vi "LIA Test CORDIC Host.vi"() -> ()   [LabVIEW 2017]
uses:
  <vilib>/userdefined/Silver/nirio_resource_slv.ctl
  <vilib>/FPGAPlugInAG/PXIe-7976R/niLvFpga_Open_PXIe-7976R.vi
  <vilib>/rvi/interface/common/dynamic/niFpgaDynamicAddResources.vi
  <vilib>/Utility/error.llb/Error Cluster From Error Code.vi
  <vilib>/rvi/errors/niLvFpgaAdjustHostInterfaceError.vi
  <vilib>/rvi/interface/common/niFpgaWaitOnOcc.vi
  <instrlib>/_niInstr/Streaming/v1/Host/Public/Start Finite Stream.vi
  <instrlib>/_niInstr/Streaming/v1/Host/Public/Wait for Stream.vi
  <vilib>/measure/maspectr.llb/FFT Power Spectrum and PSD for 1 Chan (CDB).vi
  <vilib>/FPGAPlugInAG/Dynamic/niLvFpga_Close_Dynamic.vi
  <vilib>/rvi/interface/nirviOpenFPGA/nirviOpenFPGA.xnode
  FPGA Bitfiles/LIA Test Frequency Shift.lvbitx
  <vilib>/rvi/interface/nirviReadWriteControl/nirviReadWriteControl.xnode
  <vilib>/rvi/interface/nirviMethod/nirviMethod.xnode
  <vilib>/rvi/interface/nirviCloseFPGA/nirviCloseFPGA.xnode
  <vilib>/rvi/errors/niLvFpgaMergeErrorWithErrorCode.vi
  <instrlib>/_niInstr/Streaming/v1/Host/niInstr Streaming v1 Host.lvlib
  <vilib>/rvi/interface/Simulation/niFpgaSimulationCallBeginRW.vi
  NiFpgaLv.dll
  <vilib>/measure/NI_MAPro.lvlib
  <vilib>/Analysis/NI_AALBase.lvlib
  <vilib>/FPGAPlugInAG/Dynamic/niLvFpga_StopFifo_Dynamic.vi
  <vilib>/FPGAPlugInAG/Dynamic/niLvFpga_ConfigureFifo_Dynamic.vi
  <vilib>/FPGAPlugInAG/Dynamic/niLvFpga_StartFifo_Dynamic.vi
  Program Files (x86)/National Instruments/LabVIEW 2017/examples/Lock-In Amplifier/lib/host/Lock-In Amplifier Example Host.lvlib
  <vilib>/FPGAPlugInAG/Dynamic/niLvFpga_ReadFifo_Dynamic.vi
panel:
  in  "Stop Button":bool
  in  "Output Frequency":dbl format="%#_p"
  out "standard deviation":dbl format="%0.2p"
  out "mean":dbl format="%.5p"
  out "output sample rate 0":fxp<+,48,1> format="%.48g"
  in  "Decimation":u32
  out "frequency shift rdi count":u64
  out "FIFO rdi count":u64
  in  "Frequency Shift(Hz)":dbl format="%#_p"
  out "Actual Depth":u32 format="%.0p"
  out "Power Specturm Graph":cluster{"f0":dbl, "df":dbl, "magnitude":dbl[]}[](graph)
  out "frequency shift":fxp<+/-,48,0> format="%.48g"
  out "nco frequency 0":fxp<+/-,48,0> format="%.48g"
  in  "NCO Frequency (Hz)":dbl=1000000.0 format="%#_p"
  out "Waveform Graph IQ":dbl[][](graph)
  in  "Number of Elements":u32=10000
  out "error out":errorcluster
  in  "error in":errorcluster
  in  "Resource Name":T1="PXI2Slot2"
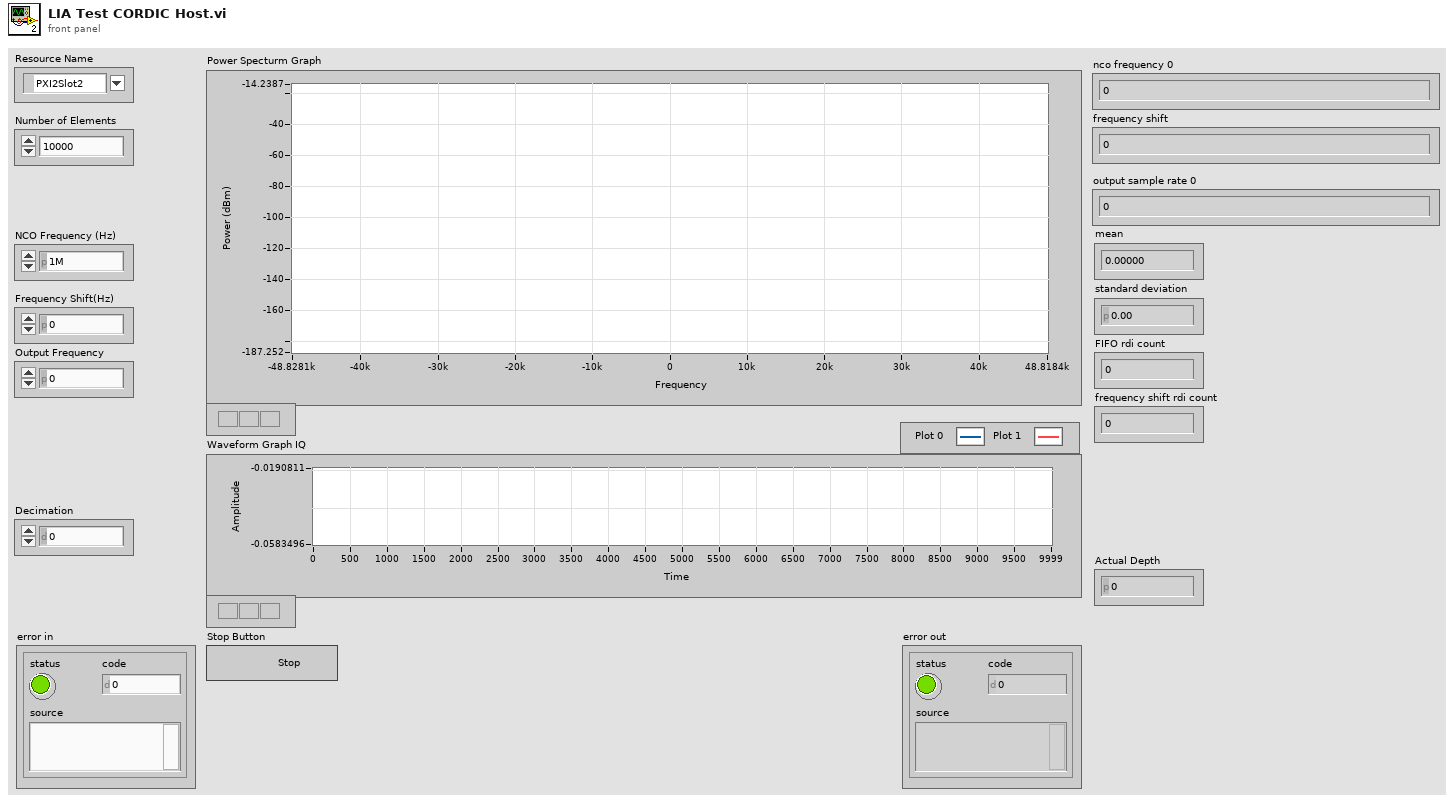
[diagram p1: front panel]
types:
  T1 = typedef "nirio_resource_slv.ctl" = tag
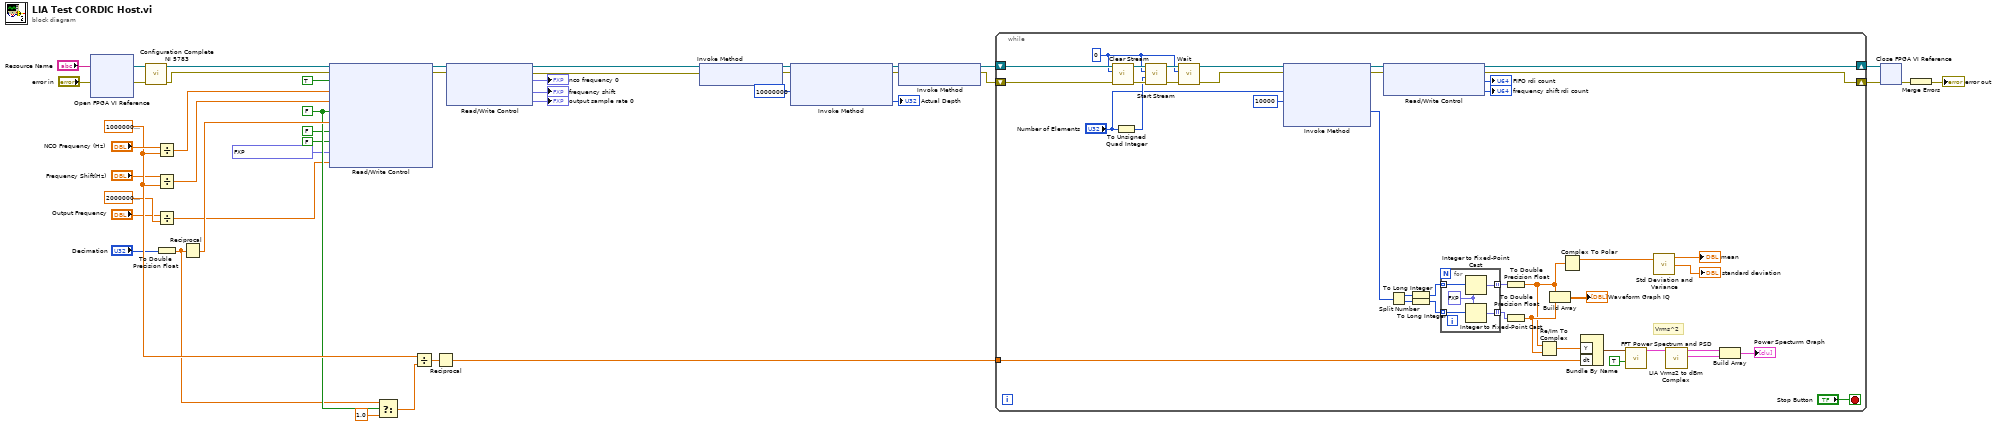
[diagram p0: block diagram]
diagram:
  w27 = 100000000.0 ("Sampling Rate (Hz)")
  w21 = FALSE ("fractional decimator 0 (F)")
  n1 = xnode "Open FPGA VI Reference"("error in"="error in", "resource name"="Resource Name") -> ("FPGA VI Reference Out"=w8:refnum<k20>, "error out"=w7:errorcluster)
  n2 = call "Configuration Complete NI 5783.vi"("error in"=w7, "fpga session in"=w8) -> ("error out"=w6:errorcluster, "fpga session out"=w5:refnum<k20>)  [unwired: 7 in, 1 out]
  n3 = Divide(x="NCO Frequency (Hz)", y=w27) -> (x/y=w39:dbl)
  n4 = Divide(x="Frequency Shift(Hz)", y=w27) -> (x/y=w14:dbl)
  n5 = Divide(x="Output Frequency", y=200000000.0) -> (x/y=w11:dbl)
  n6 = To Double Precision Float(number="Decimation") -> (double precision float=w4:dbl)
  n7 = Reciprocal(x=w4) -> (1/x=w23:dbl)
  n8 = xnode "Read/Write Control"("FPGA VI Reference In"=w5, "error in"=w6, "nco enable (T) 0"=TRUE ("nco enable (T)"), "nco frequency 0"=w39, "frequency shift 0"=w14, "fractional decimator 0 (F)"=w21, "output sample rate 0"=w23, "Select NCO? 0"=FALSE, "ao.reset 0"=FALSE, "ao.level 0"=fxp<+/-,18,1> 0.9999923706054688, "ao.carrier 0"=w11) -> ("FPGA VI Reference Out"=w10:refnum<k20>, "error out"=w3:errorcluster)
  n9 = Select(t=w4, s=w21, f=1.0) -> (s? t:f=w19:dbl)
  n10 = Divide(x=w27, y=w19) -> (x/y=w22:dbl)
  n11 = Reciprocal(x=w22) -> (1/x=w26:dbl)
  n12 = xnode "Read/Write Control"("FPGA VI Reference In"=w10, "error in"=w3) -> ("FPGA VI Reference Out"=w38:refnum<k20>, "error out"=w37:errorcluster, "nco frequency 0"=→"nco frequency 0":fxp<+/-,48,0>, "frequency shift 0"=→"frequency shift":fxp<+/-,48,0>, "output sample rate 0"=→"output sample rate 0":fxp<+,48,1>)
  n13 = xnode "Invoke Method"("FPGA VI Reference In"=w38, "error in"=w37) -> ("FPGA VI Reference Out"=w33:refnum<k20>, "error out"=w43:errorcluster)
  n14 = xnode "Invoke Method"("FPGA VI Reference In"=w33, "error in"=w43, "Requested Depth"=u32 10000000) -> ("FPGA VI Reference Out"=w32:refnum<k20>, "error out"=w34:errorcluster, "Actual Depth"=→"Actual Depth":u32)
  n15 = xnode "Invoke Method"("FPGA VI Reference In"=w32, "error in"=w34) -> ("FPGA VI Reference Out"=w2:refnum<k20>, "error out"=w1:errorcluster)
  n16 = while {
    tunnel: w26 -> [w83]
    shift-right: [w84] -> w29
    shift-left: w2 -> [w57]
    shift-right: [w85] -> w30
    shift-left: w1 -> [w56]
    stop <- "Stop Button" stop-if-true
    w46 = 0 ("stream index")
    # "Vrms^2"
    n17 = call <instrlib>:"Clear Stream.vi"("error in (no error)"=w56, "stream index"=w46, "refnum in"=w57) -> ("error out"=w54:errorcluster, "refnum out"=w55:refnum<k20>)  [unwired: 7 in]
    n18 = To Unsigned Quad Integer(1:"Number of Elements") -> (0:w49:u64)
    n19 = call-poly <instrlib>:"Start Stream.vi"("error in (no error)"=w54, "num samples"=w49, "stream index"=w46, "refnum in"=w55) -> ("error out"=w52:errorcluster, "refnum out"=w53:refnum<k20>)  [unwired: 6 in]
    n20 = call-poly <instrlib>:"Wait.vi"("error in (no error)"=w52, "stream index"=w46, "refnum in"=w53) -> ("error out"=w50:errorcluster, "refnum out"=w51:refnum<k20>)  [unwired: 5 in, 2 out]
    n21 = xnode "Invoke Method"("FPGA VI Reference In"=w51, "error in"=w50, "Number of Elements"="Number of Elements", "Timeout (ms)"=10000) -> ("FPGA VI Reference Out"=w81:refnum<k20>, "error out"=w82:errorcluster, "Data"=w67:u64[])  [unwired: 1 out]
    n22 = xnode "Read/Write Control"("FPGA VI Reference In"=w81, "error in"=w82) -> ("FPGA VI Reference Out"=w84:refnum<k20>, "error out"=w85:errorcluster, "FIFO rdi count"=→"FIFO rdi count":u64, "frequency shift rdi count"=→"frequency shift rdi count":u64)
    n23 = Split Number(x=w67) -> (hi(x)=w78:u32[], lo(x)=w77:u32[])
    n24 = To Long Integer(number=w78) -> (32bit integer=w70:i32[])
    n25 = To Long Integer(number=w77) -> (32bit integer=w69:i32[])
    n26 = for {
      tunnel: w70 -> [w90] mode=indexing
      tunnel: w69 -> [w89] mode=indexing
      tunnel: [w87] -> w76 mode=indexing
      tunnel: [w86] -> w75 mode=indexing
      w88 = fxp<+/-,18,1> 0.0 ("fixed-point type")
      n27 = Integer to Fixed-Point Cast(fixed-point type=w88, integer=w90) -> (fixed-point=w87:fxp<+/-,18,1>)
      n28 = Integer to Fixed-Point Cast(fixed-point type=w88, integer=w89) -> (fixed-point=w86:fxp<+/-,18,1>)
    }
    n29 = To Double Precision Float(number=w76) -> (double precision float=w66:dbl[])
    n30 = To Double Precision Float(number=w75) -> (double precision float=w73:dbl[])
    n31 = Re/Im To Complex(1:w73, 2:w66) -> (0:w71:cdb[])
    n32 = Build Array(w66, w73) -> (→"Waveform Graph IQ":dbl[][])
    n33 = Complex To Polar(r * e^(i*theta)=w66) -> (r=w65:dbl[])  [unwired: 1 out]
    n34 = Bundle By Name("Y"=w71, "dt"=w83) -> (w62:waveform(cdb))  [unwired: 1 in]
    n35 = call-poly <vilib>:"FFT Power Spectrum and PSD.vi"("dB On (F)"=TRUE, "time signal"=w62) -> ("Power Spectrum / PSD"=w60:cluster{"f0":dbl, "df":dbl, "magnitude":dbl[]})  [unwired: 6 in, 3 out]
    n36 = call <vilib>:"Std Deviation and Variance.vi"("X"=w65) -> ("mean"=→"mean":dbl, "standard deviation"=→"standard deviation":dbl)  [unwired: 1 in, 1 out]
    n37 = call "LIA Vrms2 to dBm Complex.vi"("Power Spectrum / PSD"=w60) -> ("output cluster"=w58:cluster{"f0":dbl, "df":dbl, "magnitude":dbl[]}, "Power Spectrum / PSD (dBm)"=w72:cluster{"f0":dbl, "df":dbl, "magnitude":dbl[]})  [unwired: 9 in]
    n38 = Build Array(w72, w58) -> (→"Power Specturm Graph":cluster{"f0":dbl, "df":dbl, "magnitude":dbl[]}[])
  }
  n39 = xnode "Close FPGA VI Reference"("FPGA VI Reference In"=w29, "error in"=w30) -> ("error out"=w42:errorcluster)
  n40 = Merge Errors(w42) -> (→"error out":errorcluster)
